vi "get_io_version.vi"(8 "error in (no error)":errorcluster, 11 "Modbus Master in":refnum<class "Modbus Master.lvclass">) -> (0 "error out":errorcluster, 2 "I/O version":string, 3 "Modbus Master out":refnum<class "Modbus Master.lvclass">)   [LabVIEW 2018]
uses:
  <vilib>/NI/Modbus Library/API/Master/Modbus Master.lvclass
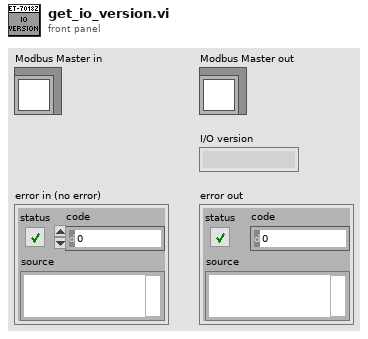
[diagram p1: front panel]
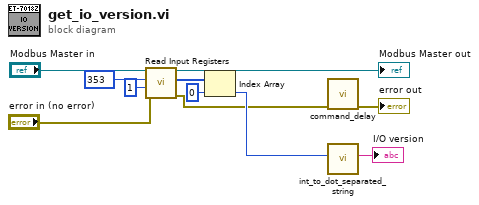
[diagram p0: block diagram]
diagram:
  n1 = call-dynamic "Read Input Registers.vi"("error in"="error in (no error)", "number of inputs"=u16 1, "starting address"=u16 353, "Modbus master in"="Modbus Master in") -> ("error out"=w1:errorcluster, "register values"=w5:u16[], "Modbus master out"=→"Modbus Master out":refnum<class "Modbus Master.lvclass">)  [unwired: 5 in]
  n2 = Index Array(array=w5, index=0) -> (element=w7:u16)
  n3 = call "command_delay.vi"("error in (no error)"=w1) -> ("error out"=→"error out":errorcluster)  [unwired: 10 in]
  n4 = call "int_to_dot_separated_string.vi"("integer"=w7) -> ("dot fmt string"=→"I/O version":string)  [unwired: 10 in]
